vi "Create.vi"(8 "error in (no error)":errorcluster, 9 "Numeric":dbl, 10 "String":string) -> (0 "error out":errorcluster, 3 "Dummy Class":refnum<class "Dummy Class.lvclass">)   [LabVIEW 2020, in "Dummy Class.lvclass"]
uses:
  Dummy Class.lvclass
  Dummy Class.lvclass/Dummy Class.ctl
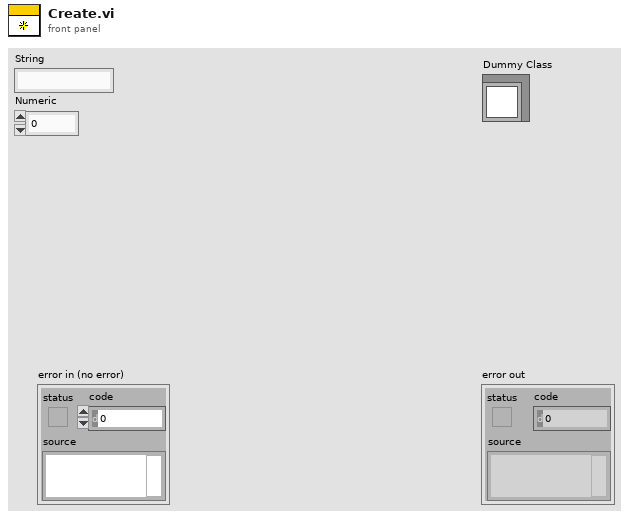
[diagram p1: front panel]
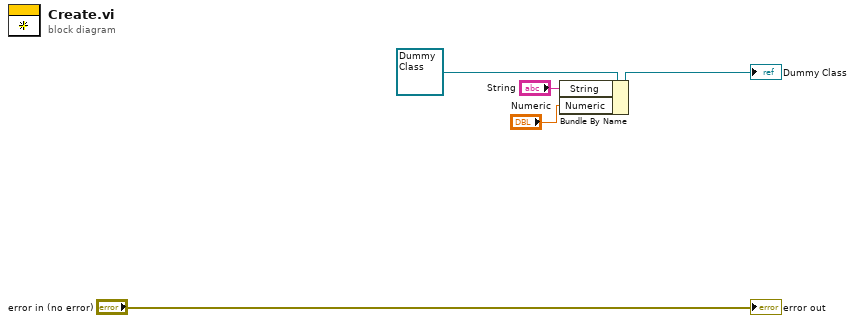
[diagram p0: block diagram]
diagram:
  n1 = Bundle By Name(cluster=refnum<class "Dummy Class.lvclass"> refnum ("Dummy Class"), "String"="String", "Numeric"="Numeric") -> (→"Dummy Class":refnum<class "Dummy Class.lvclass">)
  "error out" <- "error in (no error)"
